vi "Fetch.vi"(8 "error in (no error)":errorcluster, 11 "NISTNiPxi6123 in":refnum<class "NiPxi6123.lvclass">) -> (0 "error out":errorcluster, 3 "NISTNiPxi6123 out":refnum<class "NiPxi6123.lvclass">)   [LabVIEW 2014, in "SamplerPlugins.lvlib" / "NiPxi6123.lvclass"]
uses:
  NiPxi6123.lvclass
  <vilib>/DAQmx/read.llb/DAQmx Read (Analog 1D Wfm NChan NSamp).vi
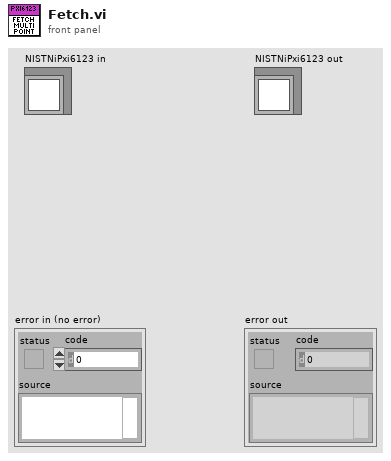
[diagram p1: front panel]
types:
  T1 = typedef "SamplerPlugins.lvlib/SamplerPluginsBase.lvclass/ReadMultiPointParams.ctl" = cluster{"iMaxTimeMilliseconds":i32, "iArraySize":i32}
  T2 = typedef "SamplerPlugins.lvlib/SamplerPluginsBase.lvclass/MultiPointReadingArrayParams.ctl" = T3[]
  T3 = typedef "SamplerPlugins.lvlib/SamplerPluginsBase.lvclass/MultiPointReadingParams.ctl" = cluster{"dReadingArray":dbl[], "iActualPts":i32, "Timestamp":dbl}
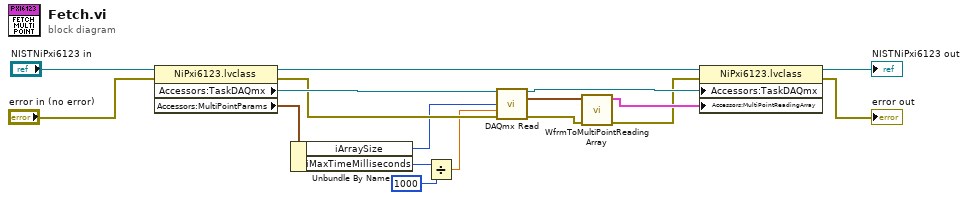
[diagram p0: block diagram]
diagram:
  n1 = property class="NiPxi6123.lvclass"(reference="NISTNiPxi6123 in", error in="error in (no error)") -> (reference out=w11:refnum<class "NiPxi6123.lvclass">, error out=w14:errorcluster, "Accessors:TaskDAQmx"=w15:refnum<k21>, "Accessors:MultiPointParams"=w16:T1)
  n2 = Unbundle By Name(w16) -> ("iArraySize"=w13:i32, "iMaxTimeMilliseconds"=w4:i32)
  n3 = Divide(x=w4, y=1000) -> (x/y=w2:dbl)
  n4 = call-poly <vilib>:"DAQmx Read.vi"("task/channels in"=w15, "number of samples per channel"=w13, "timeout"=w2, "error in"=w14) -> ("task out"=w10:refnum<k21>, "data"=w1:waveform(dbl)[], "error out"=w12:errorcluster)  [unwired: 9 in]
  n5 = call "WfrmToMultiPointReadingArray.vi"("error in (no error)"=w12, "data"=w1) -> ("error out"=w8:errorcluster, "MultiPointReadingArrayOut"=w9:T2)  [unwired: 8 in]
  n6 = property class="NiPxi6123.lvclass"(reference=w11, error in=w8, "Accessors:TaskDAQmx"=w10, "Accessors:MultiPointReadingArray"=w9) -> (reference out=→"NISTNiPxi6123 out":refnum<class "NiPxi6123.lvclass">, error out=→"error out":errorcluster)
